vi "Begin.vi"(8 "error in":errorcluster) -> (0 "error out":errorcluster)   [LabVIEW 2018]
doc: "Called before other user functions, this VI is expected to open initial I/O refnums, load in file data, and do all program initialization. Notice that the <B>error out</B> terminal is simply used for data flow. Wiring it to other structures or subVIs ensures that this VI runs first."
uses:
  Right Motors.ctl
  Left Motors.ctl
  <vilib>/Rock Robotics/WPI/Joystick/WPI_JoystickDeviceEnum.ctl
  Compressor.ctl
  Solenoids.ctl
  Controllers.ctl
  <vilib>/Rock Robotics/WPI/Utilities/WPI_GetSetVariantRefNum.vi
  <vilib>/Rock Robotics/WPI/Solenoid/WPI_SolenoidOpenSingle.vi
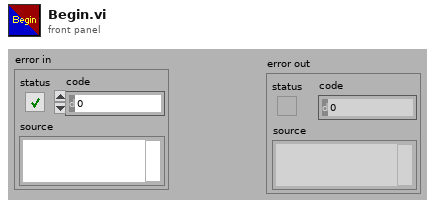
[diagram p1: front panel]
types:
  T1 = typedef "Controllers.ctl" = enum16{"Joystick 1", "Joystick 2"}
  T2 = typedef "Solenoids.ctl" = enum16{"Solenoid 1", "Solenoid 2", "Solenoid 3", "Solenoid 4"}
  T3 = typedef "Compressor.ctl" = enum16{"Compressor"}
  T4 = typedef "WPI_JoystickDeviceEnum.ctl" = enum16{"USB 0", "USB 1", "USB 2", "USB 3", "USB 4", "USB 5"}
  T5 = typedef "Left Motors.ctl" = enum16{"Left Motors 1", "Left Motors 2", "Left Motors 3"}
  T6 = typedef "Right Motors.ctl" = enum16{"Right Motors 1", "Right Motors 2", "Right Motors 3"}
  T7 = typedef "WPI_MotorControlDeviceRef.ctl" = cluster{"DeviceStatus":errorcluster, "Type":T8, "PWM":cluster{"PWM Channel":T9, "DeadBand":T10}, "CAN":cluster{"Device Number":u8, "SetOutput VI Ref":variant, "GetOutput VI Ref":variant, "Enable VI Ref":variant, "Disable VI Ref":variant, "Data":variant}, "Invert":bool, "DIO PWM":cluster{"PWM \"Enable\" Channel":T9, "DIOChannel":T11, "PWM Rate":dbl}}
  T8 = typedef "WPI_MotorControlType.ctl" = enum16{"PWM", "CAN", "DIO PWM"}
  T9 = typedef "FPGA_DIOPWMChannel.ctl" = enum8{"PWM 0", "PWM 1", "PWM 2", "PWM 3", "PWM 4", "PWM 5", "PWM 6", "PWM 7", "PWM 8", "PWM 9", "PWM MXP 0", "PWM MXP 1", "PWM MXP 2", "PWM MXP 3", "PWM MXP 4", "PWM MXP 5", "PWM MXP 6", "PWM MXP 7", "PWM MXP 8", "PWM MXP 9", "Invalid"}
  T10 = typedef "WPI_PWMDeadband.ctl" = cluster{"Name":string, "maxPositivePwm":i32, "minPositivePwm":i32, "centerPwm":i32, "maxNegativePwm":i32, "minNegativePwm":i32, "angularRange":u16}
  T11 = typedef "FPGA_DIOChannel.ctl" = enum8{"DIO 0", "DIO 1", "DIO 2", "DIO 3", "DIO 4", "DIO 5", "DIO 6", "DIO 7", "DIO 8", "DIO 9", "DIO MXP 0", "DIO MXP 1", "DIO MXP 2", "DIO MXP 3", "DIO MXP 4", "DIO MXP 5", "DIO MXP 6", "DIO MXP 7", "DIO MXP 8", "DIO MXP 9", "DIO MXP 10", "DIO MXP 11", "DIO MXP 12", "DIO MXP 13", "DIO MXP 14", "DIO MXP 15", "SPI Port CS1", "SPI Port CS2", "SPI Port CS3", "SPI Port MISO", "SPI Port MOSI", "Invalid"}
  T12 = typedef "WPI_JoystickDevRef.ctl" = cluster{"Device":T4}
  T13 = typedef "WPI_CompressorDevRef.ctl" = cluster{"DevStatus":errorcluster, "Pneumatics Control Module":u8}
  T14 = typedef "WPI_SolenoidDevRef.ctl" = cluster{"DevStatus":errorcluster, "Pneumatics Control Module":u8, "Forward Solenoid Channel":T15, "Reverse Solenoid Channel":T15}
  T15 = typedef "WPI_SolenoidChannel.ctl" = enum8{"Solenoid 0", "Solenoid 1", "Solenoid 2", "Solenoid 3", "Solenoid 4", "Solenoid 5", "Solenoid 6", "Solenoid 7", "Invalid"}
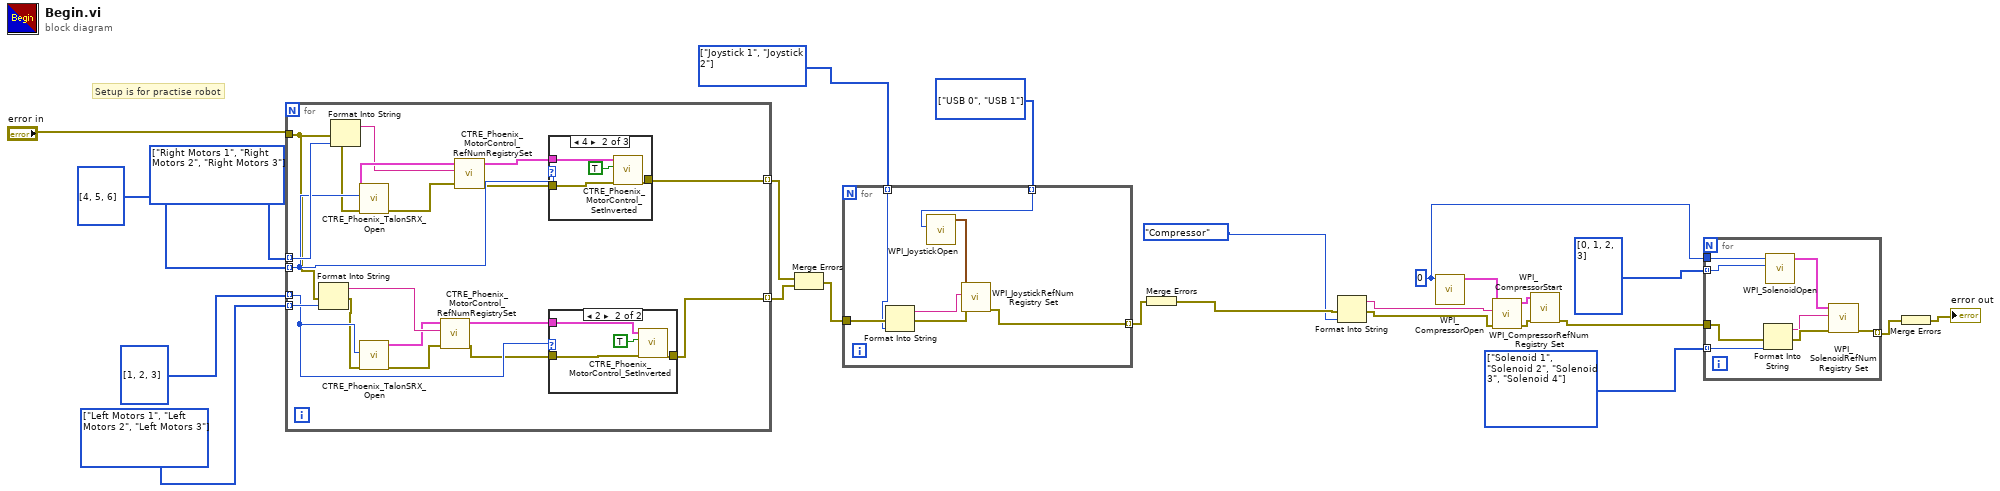
[diagram p0: block diagram]
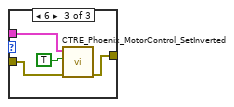
[diagram p4: hidden frame]
diagram:
  w4 = T1[] [enum."Joystick 1", enum."Joystick 2"] items=["Joystick 1", "Joystick 2"]
  w5 = T2[] [enum."Solenoid 1", enum."Solenoid 2", enum."Solenoid 3", enum."Solenoid 4"] items=["Solenoid 1", "Solenoid 2", "Solenoid 3", "Solenoid 4"]
  w9 = u8 0 ("Pneumatics Control Module (0)")
  w15 = T4[] [enum."USB 0", enum."USB 1"] items=["USB 0", "USB 1", "USB 2", "USB 3", "USB 4", "USB 5"]
  w24 = T5[] [enum."Left Motors 1", enum."Left Motors 2", enum."Left Motors 3"] items=["Left Motors 1", "Left Motors 2", "Left Motors 3"]
  w23 = T6[] [enum."Right Motors 1", enum."Right Motors 2", enum."Right Motors 3"] items=["Right Motors 1", "Right Motors 2", "Right Motors 3"]
  # "Setup is for practise robot"
  n1 = for {
    tunnel: w24 -> [w40] mode=indexing
    tunnel: w23 -> [w42] mode=indexing
    tunnel: i32[] [1, 2, 3] -> [w36] mode=indexing
    tunnel: i32[] [4, 5, 6] -> [w37] mode=indexing
    tunnel: "error in" -> [w30]
    tunnel: [w26] -> w19 mode=indexing
    tunnel: [w25] -> w18 mode=indexing
    n2 = Format Into String(error in=w30, w40) -> (resulting string=w39:string, error out=w29:errorcluster)  [unwired: 2 in]
    n3 = Format Into String(error in=w30, w42) -> (resulting string=w41:string, error out=w33:errorcluster)  [unwired: 2 in]
    n4 = call <vilib>:"CTRE_Phoenix_TalonSRX_Open.vi"("error in"=w33, "Device Number"=w37) -> ("error out"=w32:errorcluster, "CAN Talon SRX Ref"=w43:T7)  [unwired: 8 in]
    n5 = call <vilib>:"CTRE_Phoenix_TalonSRX_Open.vi"("error in"=w29, "Device Number"=w36) -> ("error out"=w28:errorcluster, "CAN Talon SRX Ref"=w38:T7)  [unwired: 8 in]
    n6 = call <vilib>:"CTRE_Phoenix_MotorControl_RefNumRegistrySet.vi"("error in (no error)"=w28, "refnum name"=w39, "PhoenixMotorControlDevRef"=w38) -> ("error out"=w27:errorcluster, "PhoenixMotorControlDevRef"=w34:T7)  [unwired: 7 in]
    n7 = call <vilib>:"CTRE_Phoenix_MotorControl_RefNumRegistrySet.vi"("error in (no error)"=w32, "refnum name"=w41, "PhoenixMotorControlDevRef"=w43) -> ("error out"=w31:errorcluster, "PhoenixMotorControlDevRef"=w35:T7)  [unwired: 7 in]
    n8 = case shown="4" w37 {
      tunnel: w35 -> [_ w53 w54]
      tunnel: w31 -> [w49 w51 w55]
      tunnel: [w49 w50 w56] -> w25
      frame Default {
      }
      frame 4 {
        n9 = call <vilib>:"CTRE_Phoenix_MotorControl_SetInverted.vi"("error in (no error)"=w51, "Invert?"=TRUE, "PhoenixMotorControlDevRef"=w53) -> ("error out"=w50:errorcluster)  [unwired: 7 in, 1 out]
      }
      frame 6 {
        n10 = call <vilib>:"CTRE_Phoenix_MotorControl_SetInverted.vi"("error in (no error)"=w55, "Invert?"=TRUE, "PhoenixMotorControlDevRef"=w54) -> ("error out"=w56:errorcluster)  [unwired: 7 in, 1 out]
      }
    }
    n11 = case shown="2" w36 {
      tunnel: w34 -> [_ w47]
      tunnel: w27 -> [w44 w46]
      tunnel: [w44 w45] -> w26
      frame Default {
      }
      frame 2 {
        n12 = call <vilib>:"CTRE_Phoenix_MotorControl_SetInverted.vi"("error in (no error)"=w46, "Invert?"=TRUE, "PhoenixMotorControlDevRef"=w47) -> ("error out"=w45:errorcluster)  [unwired: 7 in, 1 out]
      }
    }
  }
  n13 = Merge Errors(w18, w19) -> (w17:errorcluster)
  n14 = for {
    tunnel: w17 -> [w62]
    tunnel: [w60] -> w16 mode=indexing
    tunnel: w4 -> [w59] mode=indexing
    tunnel: w15 -> [w58] mode=indexing
    n15 = Format Into String(error in=w62, w59) -> (resulting string=w64:string, error out=w61:errorcluster)  [unwired: 2 in]
    n16 = call <vilib>:"WPI_JoystickOpen.vi"("JoystickDevice"=w58) -> ("JoystickDevRef"=w63:T12)  [unwired: 10 in]
    n17 = call <vilib>:"WPI_JoystickRefNum Registry Set.vi"("error in (no error)"=w61, "refnum name"=w64, "JoystickDevRef"=w63) -> ("error out"=w60:errorcluster)  [unwired: 7 in, 1 out]
  }
  n18 = Merge Errors(w16) -> (w12:errorcluster)
  n19 = Format Into String(error in=w12, Compressor."Compressor") -> (resulting string=w13:string, error out=w11:errorcluster)  [unwired: 2 in]
  n20 = call <vilib>:"WPI_CompressorOpen.vi"("Pneumatics Control Module (0)"=w9) -> ("CompressorDevRef"=w14:T13)  [unwired: 13 in, 1 out]
  n21 = call <vilib>:"WPI_CompressorRefNum Registry Set.vi"("error in (no error)"=w11, "refnum name"=w13, "CompressorDevRef"=w14) -> ("error out"=w2:errorcluster, "CompressorDevRef"=w3:T13)  [unwired: 7 in]
  n22 = call <vilib>:"WPI_CompressorStart.vi"("error in (no error)"=w2, "CompressorDevRef"=w3) -> ("error out"=w1:errorcluster)  [unwired: 8 in, 1 out]
  n23 = for {
    tunnel: w5 -> [w70] mode=indexing
    tunnel: w1 -> [w69]
    tunnel: i32[] [0, 1, 2, 3] -> [w72] mode=indexing
    tunnel: w9 -> [w71]
    tunnel: [w67] -> w7 mode=indexing
    n24 = Format Into String(error in=w69, w70) -> (resulting string=w65:string, error out=w68:errorcluster)  [unwired: 2 in]
    n25 = call-poly <vilib>:"WPI_SolenoidOpen.vi"("Solenoid Channel"=w72, "Pneumatics Control Module (0)"=w71) -> ("SolenoidDevRef"=w66:T14)  [unwired: 8 in, 1 out]
    n26 = call <vilib>:"WPI_SolenoidRefNum Registry Set.vi"("error in (no error)"=w68, "refnum name"=w65, "SolenoidDevRef"=w66) -> ("error out"=w67:errorcluster)  [unwired: 7 in, 1 out]
  }
  n27 = Merge Errors(w7) -> (→"error out":errorcluster)
